vi "init_arduino.vi"(4 "baud rate (9600)":u32=9600, 5 "Arduino's port":refnum<visa-resource-name>="COM4") -> (1 "output cluster":T1)   [LabVIEW 2015]
uses:
  <vilib>/Instr/_visa.llb/VISA Configure Serial Port (Instr).vi
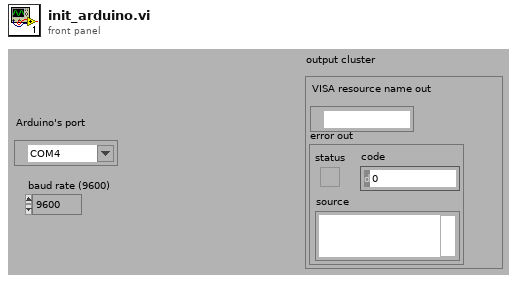
[diagram p1: front panel]
types:
  T1 = cluster{"VISA resource name out":refnum<visa-resource-name>, "error out":errorcluster}
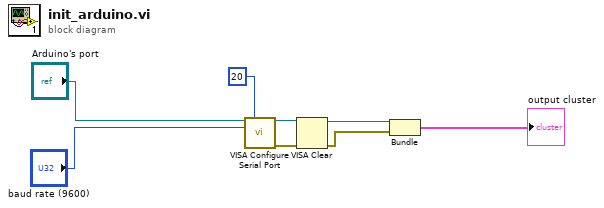
[diagram p0: block diagram]
diagram:
  n1 = call-poly "VISA Configure Serial Port"("VISA resource name"="Arduino's port", "timeout (10sec)"=u32 20, "baud rate (9600)"="baud rate (9600)") -> ("VISA resource name out"=w6:refnum<visa-resource-name>, "error out"=w5:errorcluster)  [unwired: 11 in]
  n2 = VISA Clear(VISA resource name=w6, error in (no error)=w5) -> (VISA resource name out=w4:refnum<visa-resource-name>, error out=w3:errorcluster)
  n3 = Bundle("VISA resource name out"=w4, "error out"=w3) -> (→"output cluster":T1)  [unwired: 1 in]
